vi "Scalar Addition.vi"(8 "error in (no error)":errorcluster) -> (0 "error out":errorcluster)   [LabVIEW 2023]
uses:
  <vilib>/addons/_JKI Toolkits/Caraya/classes/Test/Test.lvclass
  <vilib>/addons/_JKI Toolkits/Caraya/classes/Assert/Assert.lvclass
  SubVIs/Functions.lvlib
  <vilib>/addons/_JKI Toolkits/Caraya/classes/Assert/Assert True.vi
panel:
  # "Connector Pane"
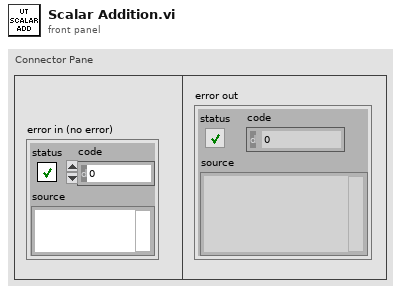
[diagram p1: front panel]
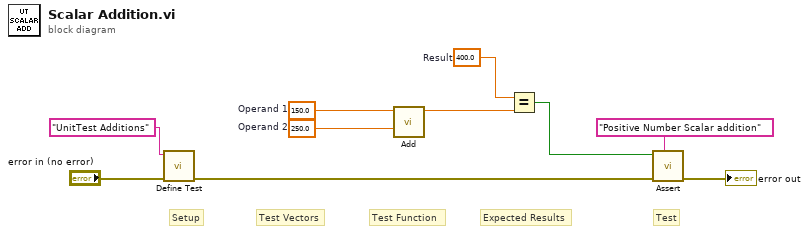
[diagram p0: block diagram]
diagram:
  w2 = 400.0  # Result
  w5 = 250.0  # Operand 2
  w6 = 150.0  # Operand 1
  # "Test Function"
  # "Expected Results"
  # "Test Vectors"
  # "Test"
  # "Setup"
  n1 = call <vilib>:"Define Test.vi"("error in (no error)"="error in (no error)", "Label (VI Title)"="UnitTest Additions") -> ("error out"=w7:errorcluster)  [unwired: 8 in, 1 out]
  n2 = call "Add.vi"("Operand 2"=w5, "Operand 1"=w6) -> ("Numeric"=w4:dbl)  [unwired: 9 in]
  n3 = Equal?(x=w2, y=w4) -> (x = y?=w3:bool)
  n4 = call-poly <vilib>:"Assert.vi"("Label"="Positive Number Scalar addition" ("Label (VI Title)"), "error in (no error)"=w7, "True?"=w3) -> ("error out"=→"error out":errorcluster)  [unwired: 7 in, 1 out]
